vi "detElementAttributes.vi"(8 "error in (no error)":errorcluster, 10 "XMLString in":string, 11 "Element in":refnum<class "XMLParser.lvclass">) -> (0 "error out":errorcluster, 3 "Element out":refnum<class "XMLParser.lvclass">)   [LabVIEW 2014, in "XML.lvlib" / "XMLParser.lvclass"]
doc: "This method calls methods from the XMLAttributeParser to extract attributes of the current element and add them to the XMLParser class data."
uses:
  <userlib>/Common/XML/XMLParser/XMLParser.lvclass
  <userlib>/Common/XML/XMLParser/XMLParser.lvclass/XMLParser.ctl
  <userlib>/Common/XML/XMLAttributeParser/XMLAttributeParser.lvclass
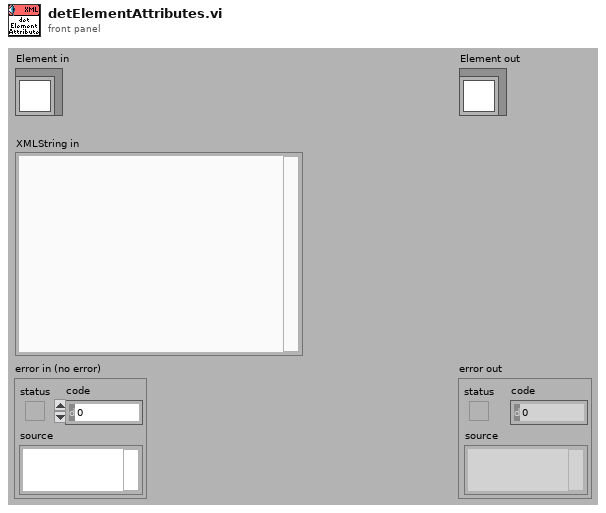
[diagram p1: front panel]
types:
  T1 = cluster{"attributeType":string, "attributeValue":string}[]
  T2 = cluster{"result string":string, "result string":string}[]
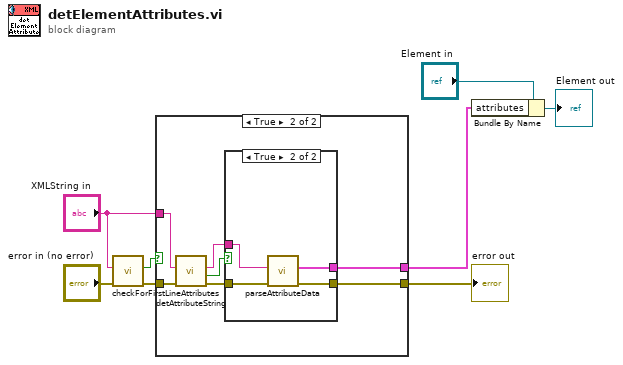
[diagram p0: block diagram]
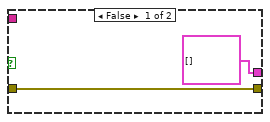
[diagram p2: hidden frame]
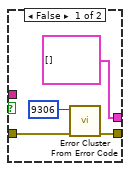
[diagram p3: hidden frame]
diagram:
  n1 = call <userlib>:"checkForFirstLineAttributes.vi"("error in (no error)"="error in (no error)", "XML In"="XMLString in") -> ("error out"=w3:errorcluster, "firstLineAttributeFound"=w2:bool)  [unwired: 7 in, 1 out]
  n2 = case shown="True" w2 {
    tunnel: [T1 [] w17] -> w8
    tunnel: [w9 w16] -> w5
    tunnel: w3 -> [w9 w12]
    tunnel: "XMLString in" -> [_ w15]
    frame False {
    }
    frame True {
      n3 = call <userlib>:"detAttributeString.vi"("error in (no error)"=w12, "XML In"=w15) -> ("error out"=w13:errorcluster, "AttributesOK?"=w11:bool, "AttributeString"=w14:string)  [unwired: 6 in, 1 out]
      n4 = case shown="True" w11 {
        tunnel: [T1 [] w25] -> w17
        tunnel: [w20 w24] -> w16
        tunnel: w14 -> [_ w23]
        tunnel: w13 -> [w21 w22]
        frame False {
          n5 = call <vilib>:"Error Cluster From Error Code.vi"("error in (no error)"=w21, "error code (0)"=9306) -> ("error out"=w20:errorcluster)  [unwired: 7 in]
        }
        frame True {
          n6 = call <userlib>:"parseAttributeData.vi"("error in (no error)"=w22, "XMLString in"=w23) -> ("error out"=w24:errorcluster, "attributeData"=w25:T2)  [unwired: 7 in, 1 out]
        }
      }
    }
  }
  "error out" <- w5
  n7 = Bundle By Name(cluster="Element in", "attributes"=w8) -> (→"Element out":refnum<class "XMLParser.lvclass">)
